vi "数据插入.vi"(8 "error in (no error)":errorcluster, 10 "table":string="铜", 11 "data":T1={"时间"=timestamp(0 s since 1904-01-01), "测量模式"="水样测试", "数据类型"="N", "检测值"=0.0, "单位"="mg/L", "数据标识"="N", "因子编码"="w20122", "标样参考值"=0.0}) -> (0 "error out":errorcluster)   [LabVIEW 2022 SP3, in "重金属.lvlib"]
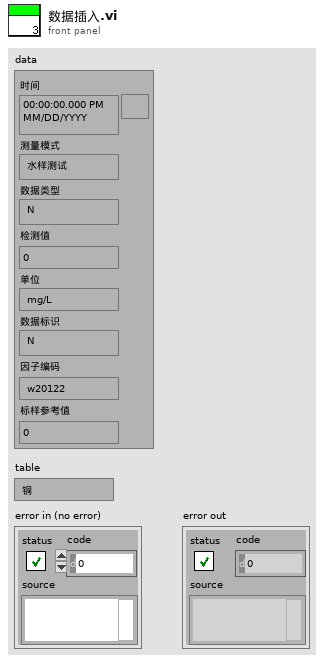
[diagram p1: front panel]
types:
  T1 = cluster{"时间":timestamp, "测量模式":string, "数据类型":string, "检测值":sgl, "单位":string, "数据标识":string, "因子编码":string, "标样参考值":sgl}
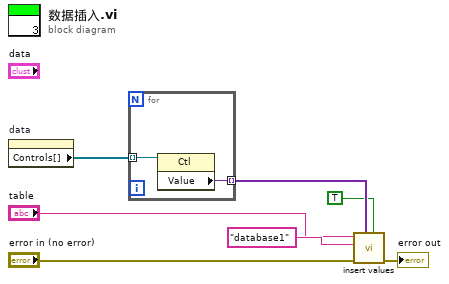
[diagram p0: block diagram]
diagram:
  n1 = property on="data" class="Clust (strict)"() -> ("Controls[]"=w7:refnum<vi>[])  [unwired: 2 in, 2 out]
  n2 = for {
    tunnel: w7 -> [w9] mode=indexing
    tunnel: [w8] -> w6 mode=indexing
    n3 = property class="Ctl"(reference=w9) -> ("Value"=w8:variant)  [unwired: 1 in, 2 out]
  }
  n4 = call "insert values.vi"("是否创建唯一键"=TRUE, "data"=w6, "错误输入（无错误）"="error in (no error)", "database"="database1", "Tabe Name"="table") -> ("错误输出"=→"error out":errorcluster)  [unwired: 6 in]
